vi "RemoveSuccessor.vi"(8 "error in (no error)":errorcluster, 10 "Node Ref":refnum<data-value>, 11 "DirectedGraphMapNode in":refnum<class "NI_Robotics_DirectedGraphMapNode.lvclass">) -> (0 "error out":errorcluster, 3 "DirectedGraphMapNode out":refnum<class "NI_Robotics_DirectedGraphMapNode.lvclass">)   [LabVIEW 2017, in "NI_Robotics_DirectedGraphMapNode.lvclass"]
uses:
  <vilib>/robotics/Navigation/shared/MapNode/DirectedGraphMapNode/NI_Robotics_DirectedGraphMapNode.lvclass
  <vilib>/robotics/Navigation/shared/MapNode/AbstractDstarNode/NI_Robotics_AbstractDstarNode.lvclass
  c:/Program Files (x86)/National Instruments/LabVIEW 2017/vi.lib/robotics/Navigation/shared/MapNode/AbstractMapNode/NI_Robotics_AbstractMapNode.lvclass
  <vilib>/robotics/Navigation/shared/MapNode/DirectedGraphMapNode/NI_Robotics_DirectedGraphMapNode.lvclass/NI_Robotics_DirectedGraphMapNode.ctl
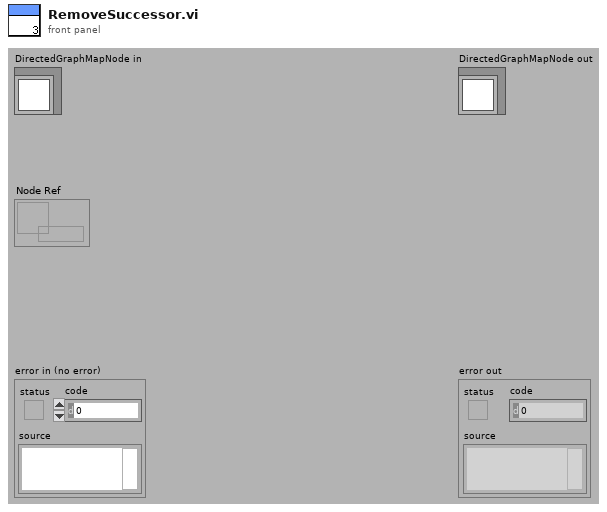
[diagram p1: front panel]
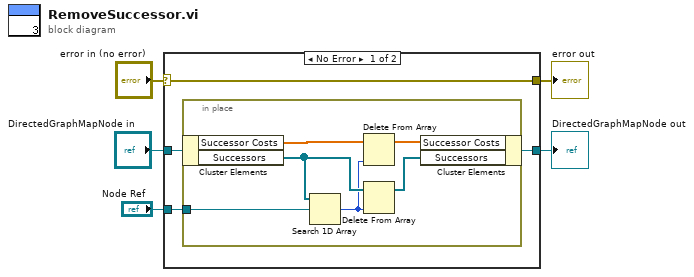
[diagram p0: block diagram]
diagram:
  n1 = case shown="No Error" "error in (no error)" {
    selector: "error in (no error)" -> [w9 w17]
    tunnel: [w9 w17] -> w4
    tunnel: [w7 w16] -> w2
    tunnel: "DirectedGraphMapNode in" -> [w8 w16]
    tunnel: "Node Ref" -> [w6 _]
    frame No Error {
      n2 = in-place {
        in-place-border: w6 -> [w15]
        n3 = in-place-cluster #1(w8) -> ("Successor Costs"=w12:dbl[], "Successors"=w14:refnum<data-value>[])
        n4 = Search 1D Array(1D array=w14, element=w15) -> (index of element=w11:i32)  [unwired: 1 in]
        n5 = Delete From Array(array=w12, index=w11) -> (array with subset deleted=w10:dbl[])  [unwired: 1 in, 1 out]
        n6 = Delete From Array(array=w14, index=w11) -> (array with subset deleted=w13:refnum<data-value>[])  [unwired: 1 in, 1 out]
        n7 = in-place-cluster #1("Successor Costs"=w10, "Successors"=w13) -> (w7:refnum<class "NI_Robotics_DirectedGraphMapNode.lvclass">)
      }
    }
    frame Error {
    }
  }
  "error out" <- w4
  "DirectedGraphMapNode out" <- w2
